vi "ENA_SettingMeas.vi"(4 "Mark_Freq(GHz)":dbl=39.0, 5 "Stop_Freq(GHz)":dbl=31.5, 6 "setSweepPoint":i32, 7 "Start_Freq(GHz)":dbl=26.5, 8 "error in":errorcluster, 9 "sParameter":i32=21, 10 "Step_Freq(GHz)":dbl=0.5 format="%#_13g", 11 "VISA IN":refnum<visa-resource-name>="TCPIP0::192.168.100.12::inst0::INSTR") -> (0 "error out":errorcluster, 3 "Marker_array":dbl[](array[numeric]))   [LabVIEW 2023, in "Keysight.lvlib"]
uses:
  CTL/Keysight_VNA.ctl
  Keysight.lvlib
panel:
  out "output cluster":T1
  in  "Mark":i32=1
  in  "Meas":i32=1
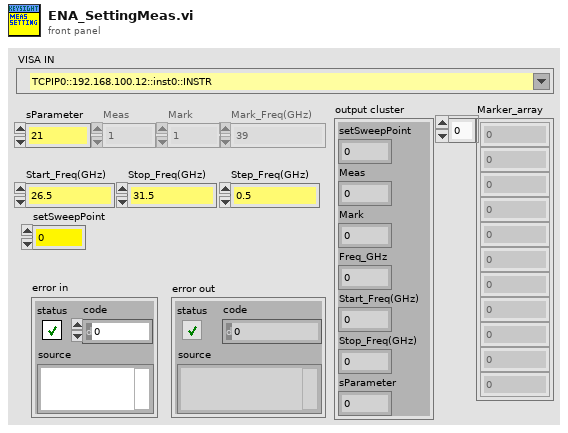
[diagram p1: front panel]
types:
  T1 = cluster{"setSweepPoint":i32, "Meas":i32, "Mark":i32, "Freq_GHz":dbl, "Start_Freq(GHz)":dbl, "Stop_Freq(GHz)":dbl, "sParameter":i32}
  T2 = typedef "Keysight_VNA.ctl" = enum16{"Init", "queryMarker", "setSweepPoint", "setMarkerFreq", "setMeasureFormat", "setFreqStartStop", "setMarkerOnOFF", "setMarkerFormat_LOGP", "setMeasPAR_S", "setTriggerSingle", "Trigger_Save_SnP", "Trigger_Single", "Close"}
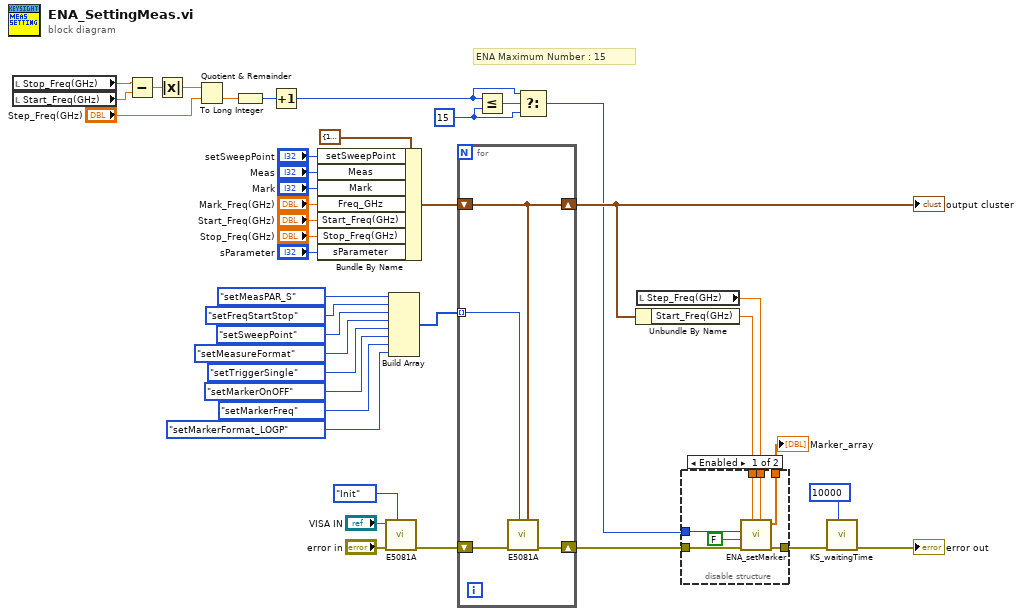
[diagram p0: block diagram]
diagram:
  w8 = 15 ("y")
  # "ENA Maximum Number : 15"
  n1 = local read "Stop_Freq(GHz)"() -> (w31:dbl)
  n2 = local read "Start_Freq(GHz)"() -> (w30:dbl)
  n3 = Subtract(x=w31, y=w30) -> (x-y=w29:dbl)
  n4 = Absolute Value(x=w29) -> (abs(x)=w27:dbl)
  n5 = Quotient & Remainder(x=w27, y="Step_Freq(GHz)") -> (floor(x/y)=w26:dbl)  [unwired: 1 out]
  n6 = To Long Integer(number=w26) -> (32bit integer=w25:i32)
  n7 = Increment(x=w25) -> (x+1=w7:i32)
  n8 = Bundle By Name(cluster=T1 {"setSweepPoint"=11, "Meas"=1, "Mark"=0, "Freq_GHz"=0.0, "Start_Freq(GHz)"=0.0, "Stop_Freq(GHz)"=0.0, "sParameter"=1} ("Input"), "setSweepPoint"="setSweepPoint", "Meas"="Meas", "Mark"="Mark", "Freq_GHz"="Mark_Freq(GHz)", "Start_Freq(GHz)"="Start_Freq(GHz)", "Stop_Freq(GHz)"="Stop_Freq(GHz)", "sParameter"="sParameter") -> (w24:T1)
  n9 = call "E5081A.vi"("Function_VNA"=Keysight_VNA."Init", "error in"="error in", "VISA IN"="VISA IN") -> ("error out"=w39:errorcluster)  [unwired: 7 in, 1 out]
  n10 = Build Array(Keysight_VNA."setMeasPAR_S" ("Function_VNA"), Keysight_VNA."setFreqStartStop" ("Function_VNA"), Keysight_VNA."setSweepPoint" ("Function_VNA"), Keysight_VNA."setMeasureFormat" ("Function_VNA"), Keysight_VNA."setTriggerSingle" ("Function_VNA"), Keysight_VNA."setMarkerOnOFF" ("Function_VNA"), Keysight_VNA."setMarkerFreq" ("Function_VNA"), Keysight_VNA."setMarkerFormat_LOGP" ("Function_VNA")) -> (w18:T2[])
  n11 = for {
    shift-right: [w44] -> w14
    shift-left: w24 -> [w44]
    tunnel: w18 -> [w43] mode=indexing
    shift-right: [w42] -> w17
    shift-left: w39 -> [w45]
    n12 = call "E5081A.vi"("Input"=w44, "Function_VNA"=w43, "error in"=w45) -> ("error out"=w42:errorcluster)  [unwired: 7 in, 1 out]
  }
  "output cluster" <- w14
  n13 = Less Or Equal?(x=w7, y=w8) -> (x <= y?=w9:bool)
  n14 = Select(t=w7, s=w9, f=w8) -> (s? t:f=w6:i32)
  n15 = Unbundle By Name(w14) -> ("Start_Freq(GHz)"=w16:dbl)
  n16 = local read "Step_Freq(GHz)"() -> (w15:dbl)
  n17 = disable-structure shown="Enabled" {
    disable-tunnel: w17 -> [w52 w53]
    disable-tunnel: w16 -> [w50 _]
    disable-tunnel: w15 -> [w49 _]
    disable-tunnel: [w48 w53] -> w13
    disable-tunnel: w6 -> [w47 _]
    disable-tunnel: [w46 _] -> w5
    frame Enabled {
      n18 = call "ENA_setMarker.vi"("Step_Freq(GHz)"=w49, "Start_Freq(GHz)"=w50, "error in"=w52, "Simulation"=FALSE, "Markers_num"=w47) -> ("error out"=w48:errorcluster, "Marker_array"=w46:dbl[])  [unwired: 5 in]
    }
    frame Disabled {
    }
  }
  "Marker_array" <- w5
  n19 = call "KS_waitingTime.vi"("Waiting Time(ms)"=u32 10000, "error in"=w13) -> ("error out"=→"error out":errorcluster)  [unwired: 9 in]
